vi "sineWaveFFT.vi"() -> ()   [LabVIEW 2015]
uses:
  <vilib>/Utility/file.llb/Read Delimited Spreadsheet (DBL).vi
  <vilib>/measure/maspectr.llb/FFT Power Spectrum and PSD for 1 Chan.vi
  <vilib>/measure/NI_MAPro.lvlib
panel:
  out "Power Spectrum / PSD":cluster{"f0":dbl, "df":dbl, "magnitude":dbl[]}(graph)
  out "output waveform":waveform(dbl)(graph)
  in  "file path":path
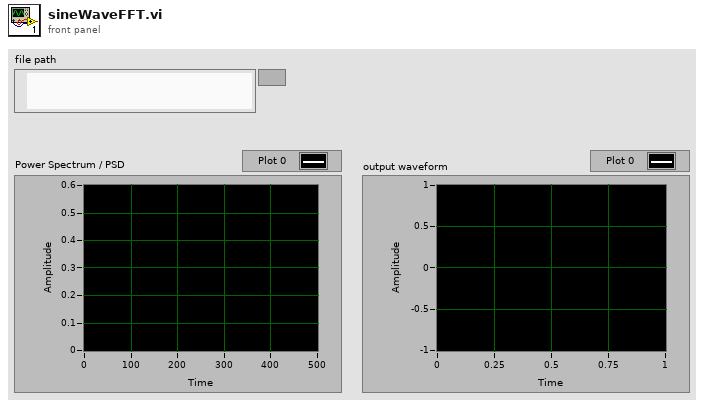
[diagram p1: front panel]
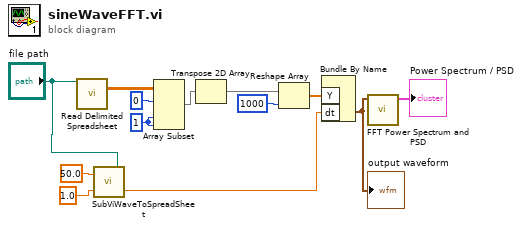
[diagram p0: block diagram]
diagram:
  w12 = 1 ("index")
  n1 = call-poly <vilib>:"Read Delimited Spreadsheet.vi"("file path (dialog if empty)"="file path") -> ("all rows"=w6:dbl[][])  [unwired: 9 in, 5 out]
  n2 = call "SubViWaveToSpreadSheet.vi"("file path (dialog if empty) 3"="file path", "amplitude"=1.0, "frequency"=50.0) -> ("dt"=w1:dbl)
  n3 = Array Subset(array=w6, index (row)=0 ("index"), index (col)=w12, length (col)=w12) -> (w11:dbl[][])  [unwired: 1 in]
  n4 = Transpose 2D Array(2D array=w11) -> (transposed array=w10:dbl[][])
  n5 = Reshape Array(w10, 1000 ("dimension size")) -> (w8:dbl[])
  n6 = Bundle By Name("Y"=w8, "dt"=w1) -> (w7:waveform(dbl))  [unwired: 1 in]
  "output waveform" <- w7
  n7 = call-poly <vilib>:"FFT Power Spectrum and PSD.vi"("time signal"=w7) -> ("Power Spectrum / PSD"=→"Power Spectrum / PSD":cluster{"f0":dbl, "df":dbl, "magnitude":dbl[]})  [unwired: 7 in, 3 out]
